vi "Read CorrectColorText.vi"(8 "error in":errorcluster, 11 "EmailField in":refnum<class "EmailField.lvclass">) -> (0 "error out":errorcluster, 2 "CorrectColorText":u32(colorbox), 3 "EmailField out":refnum<class "EmailField.lvclass">)   [LabVIEW 2020, in "EmailField.lvclass"]
uses:
  EmailField.lvclass
  EmailField.lvclass/EmailField.ctl
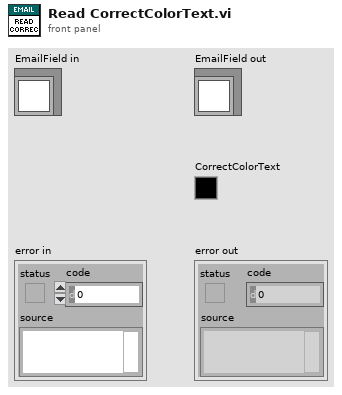
[diagram p1: front panel]
types:
  T1 = typedef "EmailField.lvclass/State Data.ctl" = cluster{"CorrectColorBG":u32, "CorrectColorText":u32, "ErrorColorBG":u32, "ErrorColorText":u32}
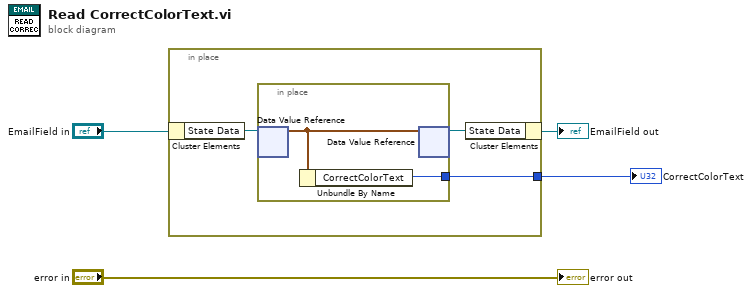
[diagram p0: block diagram]
diagram:
  n1 = in-place {
    in-place-border: [w5] -> w1
    n2 = in-place-cluster #1("EmailField in") -> ("State Data"=w7:refnum<data-value>)
    n3 = in-place {
      in-place-border: [w8] -> w5
      n4 = in-place-dvr #2(w7) -> (w9:T1)  [unwired: 1 out]
      n5 = Unbundle By Name(w9) -> ("CorrectColorText"=w8:u32)
      n6 = in-place-dvr #2(w9) -> (w6:refnum<data-value>)  [unwired: 1 out]
    }
    n7 = in-place-cluster #1("State Data"=w6) -> (→"EmailField out":refnum<class "EmailField.lvclass">)
  }
  "CorrectColorText" <- w1
  "error out" <- "error in"
